vi "get CloudComputerName.vi"(8 "error in (no error)":errorcluster caption="错误输入（无错误）") -> (0 "error out":errorcluster caption="错误输出", 3 "String/Binary data":string caption="CloudComputerName")   [LabVIEW 2016]
uses:
  <vilib>/registry/registry.llb/Registry RtKey.ctl
  <vilib>/registry/registry.llb/Registry SAM.ctl
  <vilib>/registry/registry.llb/Read Registry Value Simple STR.vi
panel:
  out "subkey":string
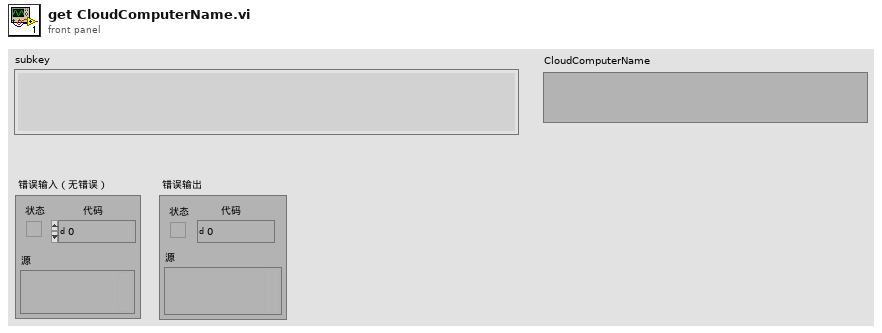
[diagram p1: front panel]
types:
  T1 = typedef "Registry SAM.ctl" = enum32{"KEY_QUERY_VALUE", "KEY_SET_VALUE", "KEY_CREATE_SUB_KEY", "KEY_ENUMERATE_SUB_KEYS", "KEY_NOTIFY", "KEY_CREATE_LINK", "KEY_READ", "KEY_WRITE", "KEY_ALL_ACCESS", "KEY_READ | KEY_WRITE"}
  T2 = typedef "Registry RtKey.ctl" = enum32{"HKEY_CLASSES_ROOT", "HKEY_CURRENT_USER", "HKEY_LOCAL_MACHINE", "HKEY_USERS", "HKEY_PERFORMANCE_DATA", "HKEY_CURRENT_CONFIG", "HKEY_DYN_DATA"}
  T3 = typedef "Registry refnum.ctl" = refnum<k1>
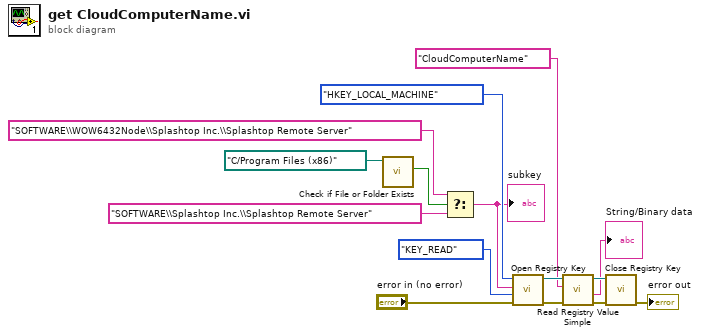
[diagram p0: block diagram]
diagram:
  n1 = call <vilib>:"Check if File or Folder Exists.vi"("path"=path "C:/Program Files (x86)") -> ("file or folder exists?"=w4:bool)  [unwired: 8 in, 2 out]
  n2 = Select(t="SOFTWARE\\WOW6432Node\\Splashtop Inc.\\Splashtop Remote Server" ("subkey"), s=w4, f="SOFTWARE\\Splashtop Inc.\\Splashtop Remote Server" ("subkey")) -> (s? t:f=w1:string)
  "subkey" <- w1
  n3 = call <vilib>:"Open Registry Key.vi"("error in (no error)"="error in (no error)", "security access mask (KEY_READ | KEY_WRITE)"=Registry_SAM."KEY_READ", "subkey"=w1, "root key (HKEY_LOCAL_MACHINE)"=Registry_RtKey."HKEY_LOCAL_MACHINE") -> ("error out"=w8:errorcluster, "refnum out"=w9:T3)  [unwired: 6 in]
  n4 = call-poly <vilib>:"Read Registry Value Simple.vi"("error in (no error)"=w8, "value"="CloudComputerName", "refnum"=w9) -> ("error out"=w13:errorcluster, "String/Binary data"=→"String/Binary data":string, "refnum out"=w14:T3)  [unwired: 3 in, 1 out]
  n5 = call <vilib>:"Close Registry Key.vi"("error in (no error)"=w13, "refnum"=w14) -> ("error out"=→"error out":errorcluster)  [unwired: 5 in]
